vi "EZDA_JS_SK.vi"() -> ()   [LabVIEW 2018]
panel:
  in  "stop":bool
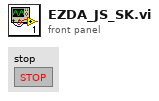
[diagram p1: front panel]
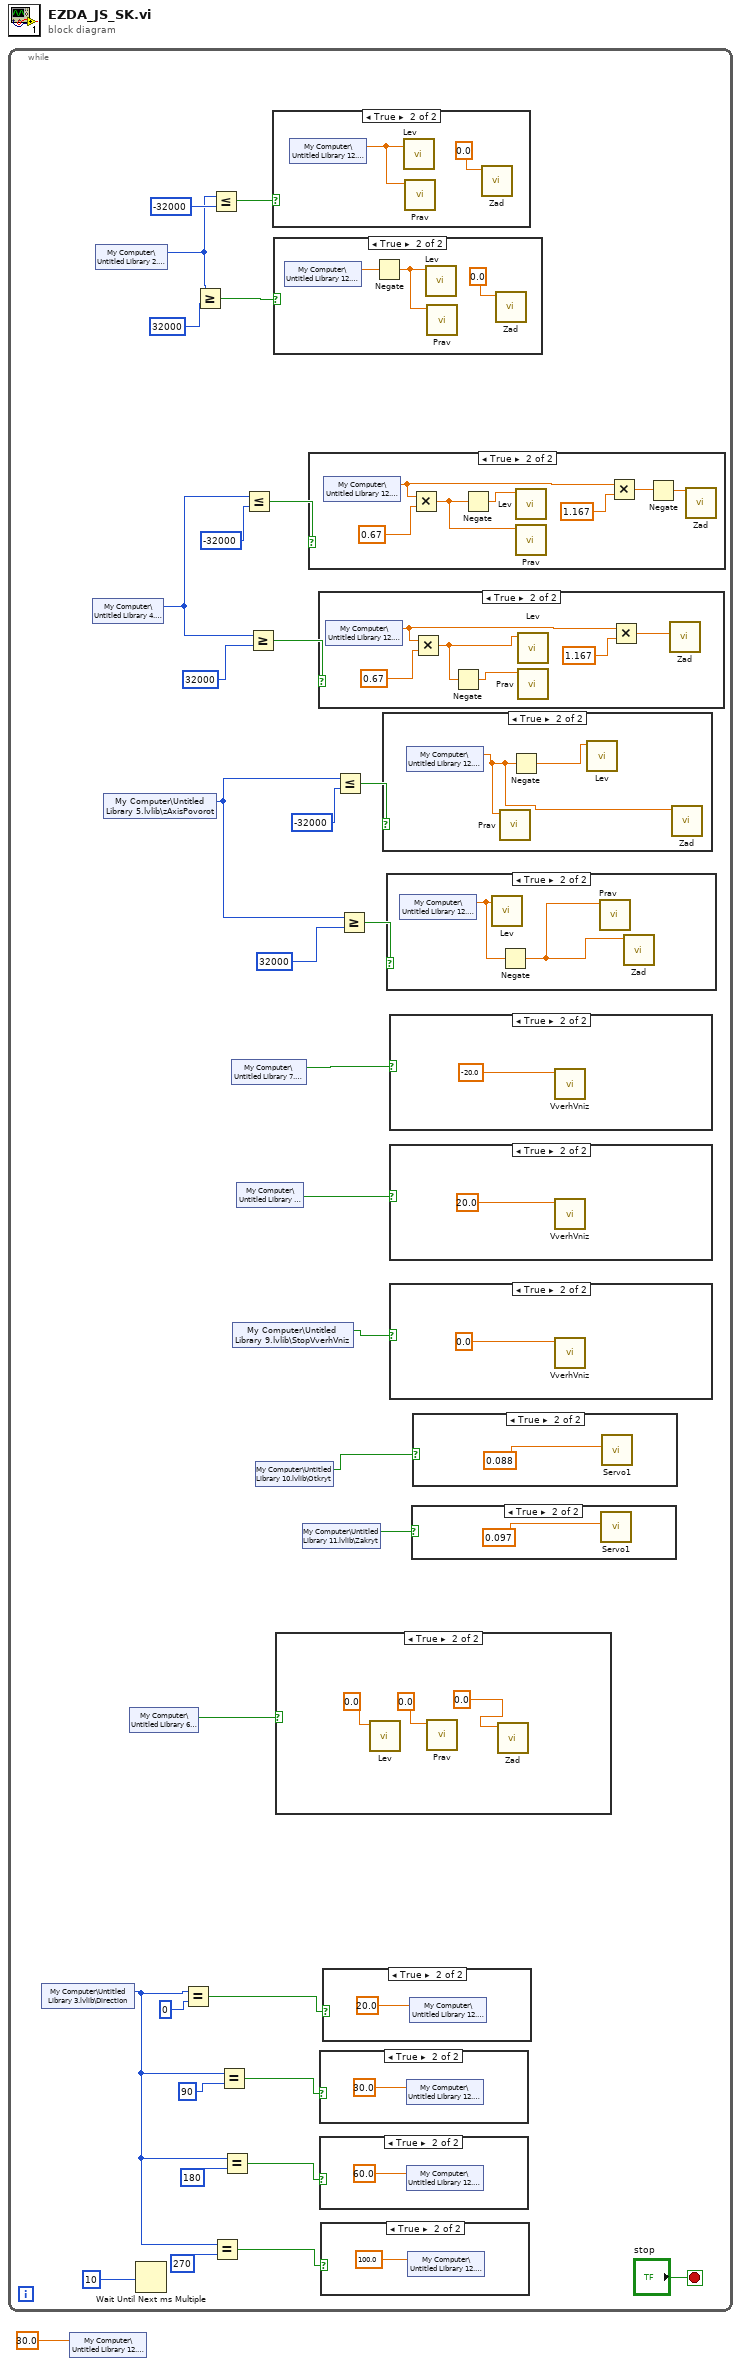
[diagram p0: block diagram]
diagram:
  n1 = while {
    stop <- "stop" stop-if-true
    n2 = shared-variable "My Computer\\Untitled Library 3.lvlib\\Direction"() -> (w3:i32)  [unwired: 1 in, 1 out]
    n3 = shared-variable "My Computer\\Untitled Library 4.lvlib\\xAxis"() -> (w22:i32)  [unwired: 1 in, 1 out]
    n4 = shared-variable "My Computer\\Untitled Library 2.lvlib\\yAxis"() -> (w27:i32)  [unwired: 1 in, 1 out]
    n5 = shared-variable "My Computer\\Untitled Library 5.lvlib\\zAxisPovorot"() -> (w17:i32)  [unwired: 1 in, 1 out]
    n6 = shared-variable "My Computer\\Untitled Library 6.lvlib\\Stop"() -> (w16:bool)  [unwired: 1 in, 1 out]
    n7 = Wait Until Next ms Multiple(millisecond multiple=10) -> ()  [unwired: 1 out]
    n8 = Equal?(x=w3, y=0) -> (x = y?=w6:bool)
    n9 = Greater Or Equal?(x=w27, y=32000) -> (x >= y?=w28:bool)
    n10 = Less Or Equal?(x=w27, y=-32000) -> (x <= y?=w32:bool)
    n11 = Equal?(x=w3, y=270) -> (x = y?=w2:bool)
    n12 = Equal?(x=w3, y=90) -> (x = y?=w5:bool)
    n13 = Equal?(x=w3, y=180) -> (x = y?=w4:bool)
    n14 = shared-variable "My Computer\\Untitled Library 7.lvlib\\Vverh"() -> (w15:bool)  [unwired: 1 in, 1 out]
    n15 = shared-variable "My Computer\\Untitled Library 9.lvlib\\StopVverhVniz"() -> (w13:bool)  [unwired: 1 in, 1 out]
    n16 = shared-variable "My Computer\\Untitled Library 8.lvlib\\Vniz"() -> (w14:bool)  [unwired: 1 in, 1 out]
    n17 = Less Or Equal?(x=w22, y=-32000) -> (x <= y?=w25:bool)
    n18 = Greater Or Equal?(x=w22, y=32000) -> (x >= y?=w23:bool)
    n19 = shared-variable "My Computer\\Untitled Library 10.lvlib\\Otkryt"() -> (w12:bool)  [unwired: 1 in, 1 out]
    n20 = case shown="True" w32 {
      frame False {
      }
      frame True {
        n21 = shared-variable "My Computer\\Untitled Library 12.lvlib\\Speed"() -> (w66:dbl)  [unwired: 1 in, 1 out]
        n22 = call "Lev.vi"("Numeric"=w66) -> ()  [unwired: 9 in, 2 out]
        n23 = call "Prav.vi"("Numeric"=w66) -> ()  [unwired: 9 in, 2 out]
        n24 = call "Zad.vi"("Numeric"=0.0) -> ()  [unwired: 9 in, 2 out]
      }
    }
    n25 = case shown="True" w28 {
      frame False {
      }
      frame True {
        n26 = shared-variable "My Computer\\Untitled Library 12.lvlib\\Speed"() -> (w64:dbl)  [unwired: 1 in, 1 out]
        n27 = Negate(x=w64) -> (-x=w63:dbl)
        n28 = call "Lev.vi"("Numeric"=w63) -> ()  [unwired: 9 in, 2 out]
        n29 = call "Prav.vi"("Numeric"=w63) -> ()  [unwired: 9 in, 2 out]
        n30 = call "Zad.vi"("Numeric"=0.0) -> ()  [unwired: 9 in, 2 out]
      }
    }
    n31 = case shown="True" w16 {
      frame False {
      }
      frame True {
        n32 = call "Lev.vi"("Numeric"=0.0) -> ()  [unwired: 9 in, 2 out]
        n33 = call "Prav.vi"("Numeric"=0.0) -> ()  [unwired: 9 in, 2 out]
        n34 = call "Zad.vi"("Numeric"=0.0) -> ()  [unwired: 9 in, 2 out]
      }
    }
    n35 = shared-variable "My Computer\\Untitled Library 11.lvlib\\Zakryt"() -> (w11:bool)  [unwired: 1 in, 1 out]
    n36 = case shown="True" w25 {
      frame False {
      }
      frame True {
        n37 = shared-variable "My Computer\\Untitled Library 12.lvlib\\Speed"() -> (w59:dbl)  [unwired: 1 in, 1 out]
        n38 = Multiply(x=w59, y=0.67) -> (x*y=w61:dbl)
        n39 = Negate(x=w61) -> (-x=w62:dbl)
        n40 = call "Lev.vi"("Numeric"=w62) -> ()  [unwired: 9 in, 2 out]
        n41 = call "Prav.vi"("Numeric"=w61) -> ()  [unwired: 9 in, 2 out]
        n42 = Multiply(x=w59, y=1.167) -> (x*y=w57:dbl)
        n43 = Negate(x=w57) -> (-x=w56:dbl)
        n44 = call "Zad.vi"("Numeric"=w56) -> ()  [unwired: 9 in, 2 out]
      }
    }
    n45 = case shown="True" w23 {
      frame False {
      }
      frame True {
        n46 = shared-variable "My Computer\\Untitled Library 12.lvlib\\Speed"() -> (w54:dbl)  [unwired: 1 in, 1 out]
        n47 = Multiply(x=w54, y=0.67) -> (x*y=w52:dbl)
        n48 = Negate(x=w52) -> (-x=w51:dbl)
        n49 = call "Lev.vi"("Numeric"=w52) -> ()  [unwired: 9 in, 2 out]
        n50 = call "Prav.vi"("Numeric"=w51) -> ()  [unwired: 9 in, 2 out]
        n51 = Multiply(x=w54, y=1.167) -> (x*y=w50:dbl)
        n52 = call "Zad.vi"("Numeric"=w50) -> ()  [unwired: 9 in, 2 out]
      }
    }
    n53 = case shown="True" w5 {
      frame False {
      }
      frame True {
        n54 = shared-variable "My Computer\\Untitled Library 12.lvlib\\Speed"(30.0) -> ()  [unwired: 1 in, 1 out]
      }
    }
    n55 = case shown="True" w4 {
      frame False {
      }
      frame True {
        n56 = shared-variable "My Computer\\Untitled Library 12.lvlib\\Speed"(60.0) -> ()  [unwired: 1 in, 1 out]
      }
    }
    n57 = case shown="True" w2 {
      frame False {
      }
      frame True {
        n58 = shared-variable "My Computer\\Untitled Library 12.lvlib\\Speed"(100.0) -> ()  [unwired: 1 in, 1 out]
      }
    }
    n59 = case shown="True" w6 {
      frame False {
      }
      frame True {
        n60 = shared-variable "My Computer\\Untitled Library 12.lvlib\\Speed"(20.0) -> ()  [unwired: 1 in, 1 out]
      }
    }
    n61 = Less Or Equal?(x=w17, y=-32000) -> (x <= y?=w20:bool)
    n62 = Greater Or Equal?(x=w17, y=32000) -> (x >= y?=w18:bool)
    n63 = case shown="True" w20 {
      frame False {
      }
      frame True {
        n64 = shared-variable "My Computer\\Untitled Library 12.lvlib\\Speed"() -> (w48:dbl)  [unwired: 1 in, 1 out]
        n65 = call "Prav.vi"("Numeric"=w48) -> ()  [unwired: 9 in, 2 out]
        n66 = Negate(x=w48) -> (-x=w49:dbl)
        n67 = call "Lev.vi"("Numeric"=w49) -> ()  [unwired: 9 in, 2 out]
        n68 = call "Zad.vi"("Numeric"=w48) -> ()  [unwired: 9 in, 2 out]
      }
    }
    n69 = case shown="True" w18 {
      frame False {
      }
      frame True {
        n70 = shared-variable "My Computer\\Untitled Library 12.lvlib\\Speed"() -> (w46:dbl)  [unwired: 1 in, 1 out]
        n71 = call "Lev.vi"("Numeric"=w46) -> ()  [unwired: 9 in, 2 out]
        n72 = Negate(x=w46) -> (-x=w47:dbl)
        n73 = call "Prav.vi"("Numeric"=w47) -> ()  [unwired: 9 in, 2 out]
        n74 = call "Zad.vi"("Numeric"=w47) -> ()  [unwired: 9 in, 2 out]
      }
    }
    n75 = case shown="True" w15 {
      frame False {
      }
      frame True {
        n76 = call "VverhVniz.vi"("Numeric"=-20.0) -> ()  [unwired: 10 in, 1 out]
      }
    }
    n77 = case shown="True" w14 {
      frame False {
      }
      frame True {
        n78 = call "VverhVniz.vi"("Numeric"=20.0) -> ()  [unwired: 10 in, 1 out]
      }
    }
    n79 = case shown="True" w13 {
      frame False {
      }
      frame True {
        n80 = call "VverhVniz.vi"("Numeric"=0.0) -> ()  [unwired: 10 in, 1 out]
      }
    }
    n81 = case shown="True" w11 {
      frame False {
      }
      frame True {
        n82 = call "Servo1.vi"("Knob"=0.097) -> ()  [unwired: 10 in, 1 out]
      }
    }
    n83 = case shown="True" w12 {
      frame False {
      }
      frame True {
        n84 = call "Servo1.vi"("Knob"=0.088) -> ()  [unwired: 10 in, 1 out]
      }
    }
  }
  n85 = shared-variable "My Computer\\Untitled Library 12.lvlib\\Speed"(30.0) -> ()  [unwired: 1 in, 1 out]
